vi "nD Nonlinear System Solver (Formula).vi"(5 "accuracy":dbl=1e-08 format="%0.2e", 6 "F(X)":string[](array[string]), 7 "number of trials":u32=5, 8 "X":string[](array[string]), 9 "End":dbl[](array[numeric]) format="%0.2f", 10 "Start":dbl[](array[numeric]) format="%0.2f", 11 "h":dbl=1e-08 format="%0.2e") -> (0 "error":i32, 1 "ticks":u32, 2 "f(Zeroes)":dbl[][](array[numeric]) format="%0.2e", 3 "Zeroes":dbl[][](array[numeric]) format="%0.2e")   [LabVIEW 2010, in "NI_Gmath.lvlib"]
doc: "Determines a set of solutions of a nonlinear system of equations in n dimensions beginning with a randomly chosen start point in n dimensions. You must manually select the polymorphic instance to use."
uses:
  NI_Gmath.lvlib
panel:
  out "error message":string="input OK!"
  out "error text":string[](array[string])
  out "error code":i32[](array[numeric])
  # "Example:\n\n accuracy: 1E-8 \n number of trials: 5 \n h: 1E-8 \n Start: 0.0 and 0.0\n End: 1.0 and 1.0\n X: x and y\n F(X): sin(x+y) and cos(x-y)"
  # "error information"
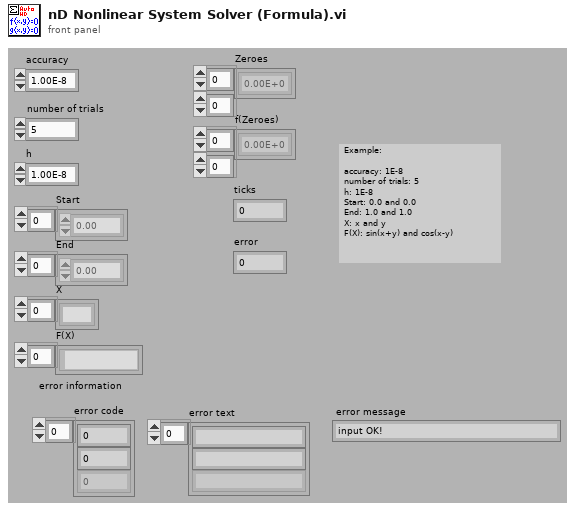
[diagram p1: front panel]
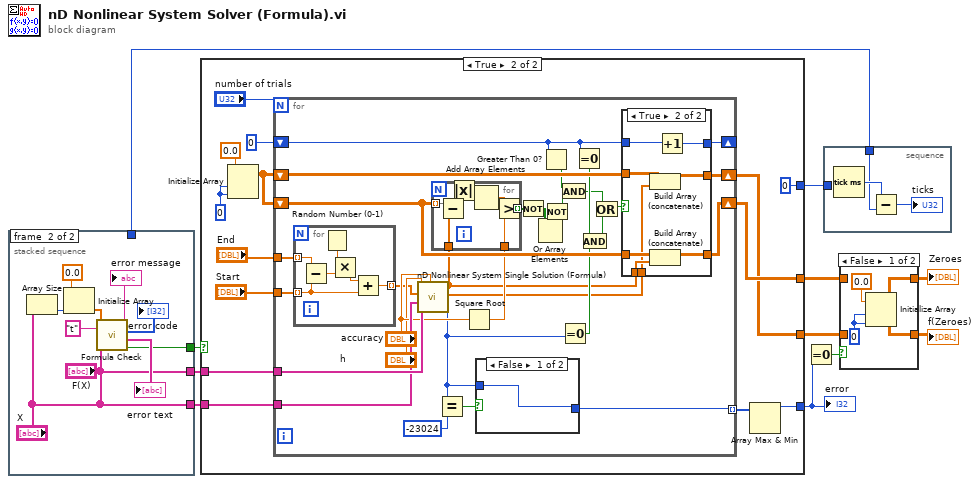
[diagram p0: block diagram]
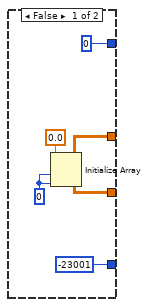
[diagram p3: hidden frame]
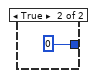
[diagram p4: hidden frame]
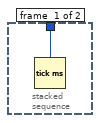
[diagram p6: hidden frame]
diagram:
  n1 = stacked-sequence {
    tunnel: [_ w15] -> w11
    tunnel: [w12 _] -> w9
    tunnel: [_ "X"] -> w8
    tunnel: [_ "F(X)"] -> w7
    frame #0 {
      n2 = Tick Count (ms)() -> (millisecond timer value=w12:u32)
    }
    frame #1 {
      n3 = Array Size(array="X") -> (size(s)=w20:i32)
      n4 = Initialize Array(0.0, w20) -> (w22:dbl[])
      n5 = call "Formula Check.vi"("F(X,t)"="F(X)", "X"="X", "time"="t", "X(0)"=w22) -> ("system error"=w15:bool, "error text"=→"error text":string[], "error"=→"error code":i32[], "error message"=→"error message":string)  [unwired: 4 out]
    }
  }
  n6 = case shown="True" w11 {
    tunnel: [0 0] -> w10
    tunnel: w8 -> [_ w38]
    tunnel: w7 -> [_ w37]
    tunnel: [w23 w32] -> w6
    tunnel: [w23 w31] -> w4
    tunnel: [-23001 w28] -> w2
    frame False {
      w24 = 0
      n7 = Initialize Array(0.0, w24, w24) -> (w23:dbl[][])
    }
    frame True {
      w34 = 0
      n8 = Initialize Array(0.0, w34, w34) -> (w35:dbl[][])
      n9 = for {
        N: "number of trials" -> [_]
        tunnel: "End" -> [w71]
        tunnel: "Start" -> [w70]
        tunnel: w38 -> [w64]
        tunnel: w37 -> [w65]
        shift-right: [w51] -> w31
        shift-left: w35 -> [w57]
        shift-right: [w52] -> w32
        shift-left: w35 -> [w68]
        tunnel: [w58] -> w30 mode=indexing
        shift-right: [w56] -> _
        shift-left: 0 -> [w47]
        n10 = for {
          tunnel: w71 -> [w97] mode=indexing
          tunnel: w70 -> [w94] mode=indexing
          tunnel: [w92] -> w61 mode=indexing
          n11 = Subtract(x=w97, y=w94) -> (x-y=w96:dbl)
          n12 = Random Number (0-1)() -> (number: 0 to 1=w95:dbl)
          n13 = Multiply(x=w95, y=w96) -> (x*y=w93:dbl)
          n14 = Add(x=w93, y=w94) -> (x+y=w92:dbl)
        }
        n15 = call "nD Nonlinear System Single Solution (Formula).vi"("accuracy"="accuracy", "F(X)"=w65, "X"=w64, "Start"=w61, "h"="h") -> ("error"=w45:i32, "f(Zeroes)"=w46:dbl[], "Zeroes"=w44:dbl[])  [unwired: 4 out]
        n16 = Equal?(x=w45, y=-23024) -> (x = y?=w59:bool)
        n17 = Square Root(x="accuracy") -> (sqrt(x)=w66:dbl)
        n18 = for {
          tunnel: w68 -> [w91] mode=indexing
          tunnel: w44 -> [w90]
          tunnel: [w86] -> w69 mode=indexing
          tunnel: w66 -> [w87]
          n19 = Subtract(x=w91, y=w90) -> (x-y=w89:dbl[])
          n20 = Absolute Value(x=w89) -> (abs(x)=w88:dbl[])
          n21 = Add Array Elements(numeric array=w88) -> (sum=w85:dbl)
          n22 = Greater?(x=w85, y=w87) -> (0:w86:bool)
        }
        n23 = case shown="False" w59 {
          tunnel: [w72 0] -> w58
          tunnel: w45 -> [w72 _]
          frame False {
          }
          frame True {
          }
        }
        n24 = Not(x=w69) -> (.not. x?=w43:bool[])
        n25 = Or Array Elements(Boolean array=w43) -> (logical OR=w49:bool)
        n26 = Greater Than 0?(x=w47) -> (x > 0?=w50:bool)
        n27 = Not(x=w49) -> (.not. x?=w42:bool)
        n28 = And(x=w50, y=w42) -> (x .and. y?=w48:bool)
        n29 = Equal To 0?(x=w45) -> (x = 0?=w54:bool)
        n30 = Equal To 0?(x=w47) -> (x = 0?=w53:bool)
        n31 = And(x=w53, y=w54) -> (x .and. y?=w55:bool)
        n32 = Or(x=w48, y=w55) -> (x .or. y?=w67:bool)
        n33 = case shown="True" w67 {
          tunnel: w57 -> [w76 w80]
          tunnel: [w76 w79] -> w51
          tunnel: w68 -> [w75 w83]
          tunnel: [w75 w82] -> w52
          tunnel: w44 -> [_ w84]
          tunnel: w46 -> [_ w81]
          tunnel: w47 -> [w74 w78]
          tunnel: [w74 w77] -> w56
          frame False {
          }
          frame True {
            n34 = Build Array (concatenate)(w80, w81) -> (w79:dbl[][])
            n35 = Build Array (concatenate)(w83, w84) -> (w82:dbl[][])
            n36 = Increment(x=w78) -> (x+1=w77:i32)
          }
        }
      }
      n37 = Array Max & Min(array=w30) -> (max value=w28:i32)  [unwired: 3 out]
    }
  }
  "error" <- w2
  n38 = Equal To 0?(x=w2) -> (x = 0?=w1:bool)
  n39 = stacked-sequence {
    tunnel: w9 -> [w99]
    tunnel: w10 -> [_]
    frame #0 {
      n40 = Tick Count (ms)() -> (millisecond timer value=w100:u32)
      n41 = Subtract(x=w100, y=w99) -> (x-y=→"ticks":u32)
    }
  }
  n42 = case shown="False" w1 {
    tunnel: w6 -> [_ w105]
    tunnel: [w101 w105] -> w5
    tunnel: w4 -> [_ w104]
    tunnel: [w101 w104] -> w3
    frame False {
      w103 = 0
      n43 = Initialize Array(0.0, w103, w103) -> (w101:dbl[][])
    }
    frame True {
    }
  }
  "Zeroes" <- w5
  "f(Zeroes)" <- w3
